vi "VNA Configuration - SParam.vi"(8 "error in":errorcluster, 10 "RFmxVNA Settings":T1={"Resource Name"="", "vCal Name"="", "RFmxVNA Calset Enable"=FALSE, "RFmxVNA Calset Interpolation"=FALSE, "Calset File Path"="", "RFmxVNA attenuation mode"=enum."s2p File", "RFmxVNA Port1 s2p file path"="", "RFmxVNA Port1 s-parameters orientation"=enum."Port1 Towards DUT", "RFmxVNA Port1 Power Compensation"=FALSE, "RFmxVNA Port2 s2p file path"="", "RFmxVNA Port2 s-parameters orientation"=enum."Port1 Towards DUT", "RFmxVNA Port2 Power Compensation"=FALSE, "Port1 Power Level (dBm)"=0.0, "Port1 Test Receiver Attenuation (dB)"=0.0, "Port2 Power Level (dBm)"=0.0, "Port2 Test Receiver Attenuation (dB)"=0.0, "IF Bandwidth (Hz)"=0.0, "Frequency Sweep"={"Start Frequency (Hz)"=4000000000.0, "Stop Frequency (Hz)"=26000000000.0, "Number of Points"=200}} {"Frequency Sweep"."Stop Frequency (Hz)" format="%.3p"; "Frequency Sweep"."Start Frequency (Hz)" format="%.3p"; "IF Bandwidth (Hz)" format="%.2p"; "Port2 Test Receiver Attenuation (dB)" format="%.2f"; "Port2 Power Level (dBm)" format="%.2f"; "Port1 Test Receiver Attenuation (dB)" format="%.2f"; "Port1 Power Level (dBm)" format="%.2f"}, 11 "RFmxVNA Session in":refnum<k21>) -> (0 "error out":errorcluster, 3 "RFmxVNA Session out":refnum<k21>)   [LabVIEW 2023]
uses:
  <resource>/objmgr/RFmxVNA.rc
  Controls/RFmxVNA Config - SParam.ctl
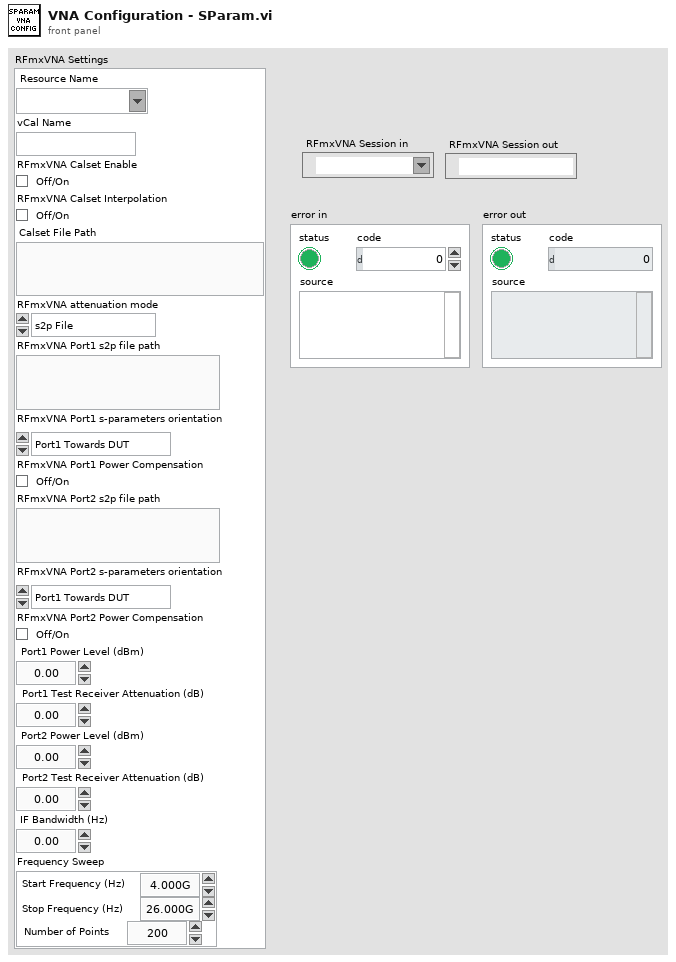
[diagram p1: front panel]
types:
  T1 = typedef "RFmxVNA Config - SParam.ctl" = cluster{"Resource Name":refnum<k15>, "vCal Name":string, "RFmxVNA Calset Enable":bool, "RFmxVNA Calset Interpolation":bool, "Calset File Path":string, "RFmxVNA attenuation mode":enum32{"<None>", "s2p File"}, "RFmxVNA Port1 s2p file path":string, "RFmxVNA Port1 s-parameters orientation":enum32{"Port1 Towards DUT", "Port2 Towards DUT"}, "RFmxVNA Port1 Power Compensation":bool, "RFmxVNA Port2 s2p file path":string, "RFmxVNA Port2 s-parameters orientation":enum32{"Port1 Towards DUT", "Port2 Towards DUT"}, "RFmxVNA Port2 Power Compensation":bool, "Port1 Power Level (dBm)":dbl, "Port1 Test Receiver Attenuation (dB)":dbl, "Port2 Power Level (dBm)":dbl, "Port2 Test Receiver Attenuation (dB)":dbl, "IF Bandwidth (Hz)":dbl, "Frequency Sweep":cluster{"Start Frequency (Hz)":dbl, "Stop Frequency (Hz)":dbl, "Number of Points":i32}}
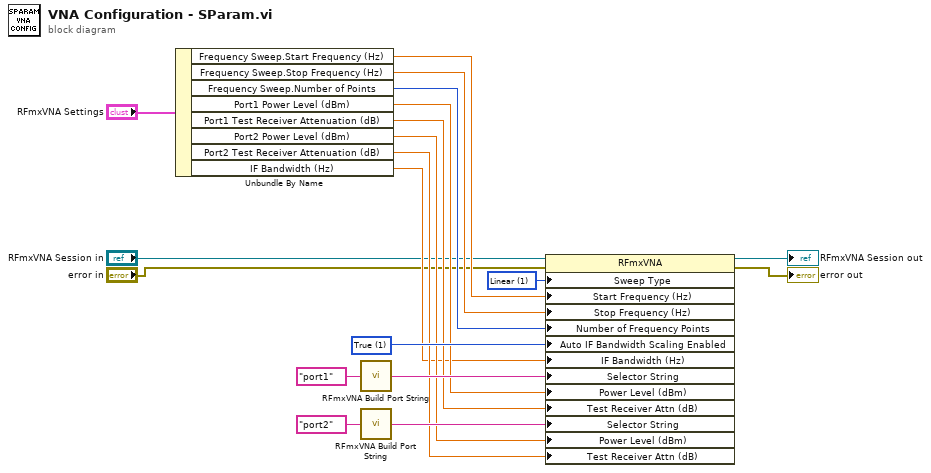
[diagram p0: block diagram]
diagram:
  w14 = 1 items=["List", "Linear", "Segment"] ("Sweep Type")
  w19 = 1 items=["False", "True"] ("Auto IF Bandwidth Scaling Enabled")
  n1 = Unbundle By Name("RFmxVNA Settings") -> ("Frequency Sweep.Start Frequency (Hz)"=w12:dbl, "Frequency Sweep.Stop Frequency (Hz)"=w11:dbl, "Frequency Sweep.Number of Points"=w10:i32, "Port1 Power Level (dBm)"=w9:dbl, "Port1 Test Receiver Attenuation (dB)"=w8:dbl, "Port2 Power Level (dBm)"=w7:dbl, "Port2 Test Receiver Attenuation (dB)"=w6:dbl, "IF Bandwidth (Hz)"=w5:dbl)
  n2 = call <vilib>:"RFmxVNA Build Port String.vi"("Port Name"="port1" ("Port")) -> ("Selector String Out"=w16:string)  [unwired: 14 in]
  n3 = call <vilib>:"RFmxVNA Build Port String.vi"("Port Name"="port2" ("Port")) -> ("Selector String Out"=w17:string)  [unwired: 14 in]
  n4 = property class="RFmxVNA"(reference="RFmxVNA Session in", error in="error in", "Sweep Type"=w14, "Start Frequency (Hz)"=w12, "Stop Frequency (Hz)"=w11, "Number of Frequency Points"=w10, "Auto IF Bandwidth Scaling Enabled"=w19, "IF Bandwidth (Hz)"=w5, "Selector String"=w16, "Power Level (dBm)"=w9, "Test Receiver Attn (dB)"=w8, "Selector String"=w17, "Power Level (dBm)"=w7, "Test Receiver Attn (dB)"=w6) -> (reference out=→"RFmxVNA Session out":refnum<k21>, error out=→"error out":errorcluster)
